vi "R to T.vi"(7 "Resistance (Ohm)":dbl=10000.0 format="%.2f") -> (8 "Temp (deg C)":dbl=25.793583992402546 format="%.2f")   [LabVIEW 2016]
doc: "This subvi converts from resistance to temperature using the Steinhart-Hart equation for a 10 KOhm NTC thermistor. These values are only approximate without calibration. The exact parameters vary from thermistor to thermistor and need to be entered for the specific thermsitor being used. The calibration data will be supplied by your instructor. \n\nPaul K Dixon\nP350\nCSUSB Physics"
panel:
  out "Temp (deg K)":dbl=298.9435839924025 format="%.2f"
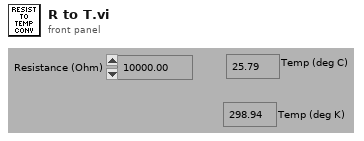
[diagram p1: front panel]
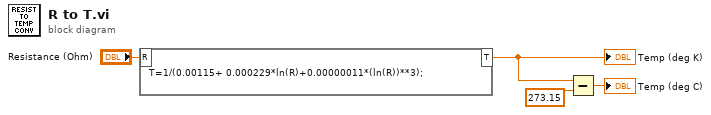
[diagram p0: block diagram]
diagram:
  n1 = formula code="T=1/(0.00115+ 0.000229*ln(R)+0.00000011*(ln(R))**3);"("R"="Resistance (Ohm)") -> ("T"=w3:dbl)
  "Temp (deg K)" <- w3
  n2 = Subtract(x=w3, y=273.15) -> (x-y=→"Temp (deg C)":dbl)
